vi "Destroy User Event - Stop.vi"(8 "error in (no error)":errorcluster, 11 "DNL_User Event - Stop":refnum<user-event>) -> (0 "error out":errorcluster)   [LabVIEW 2011, in "User Event - Stop.lvlib"]
doc: "Destroy the user event, even if there is an incoming error."
uses:
  User Event - Stop.lvlib
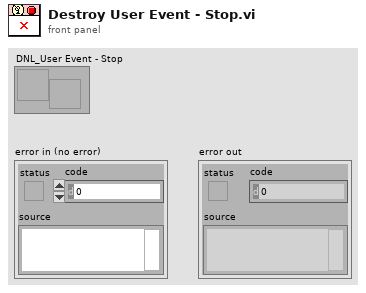
[diagram p1: front panel]
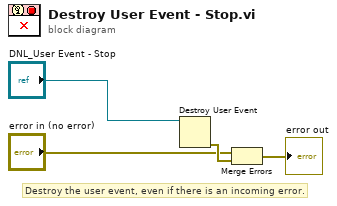
[diagram p0: block diagram]
diagram:
  # "Destroy the user event, even if there is an incoming error."
  n1 = Destroy User Event(user event="DNL_User Event - Stop") -> (error out=w3:errorcluster)  [unwired: 1 in]
  n2 = Merge Errors("error in (no error)", w3) -> (→"error out":errorcluster)
